vi "_is.vi"(8 "error in (no error)":errorcluster, 11 "Config Plugin in":refnum<class "Config Plugin.lvclass">) -> (0 "error out":errorcluster, 3 "Config Plugin out":refnum<class "Config Plugin.lvclass">)   [LabVIEW 2016, in "Config Plugin.lvlib" / "Config Plugin.lvclass"]
uses:
  <userlib>/Common Components/Config Plugin/Config Plugin.lvclass
panel:
  out "type":string
  # "HW Controller: always shown.\nspecific HW: shown when the hardware class is loaded.\nAbstract Class: for this root class"
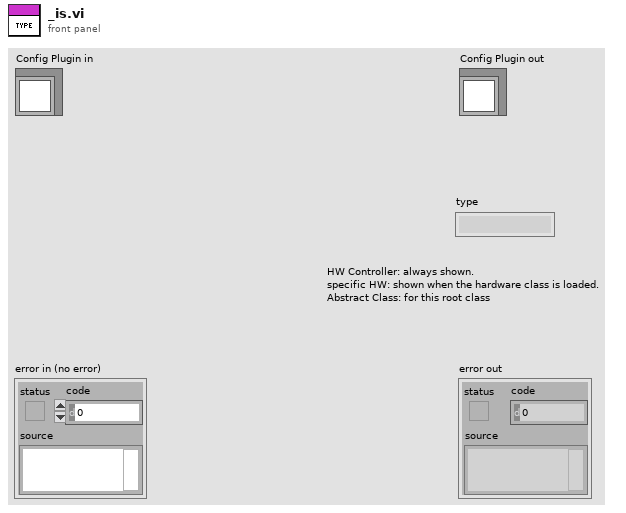
[diagram p1: front panel]
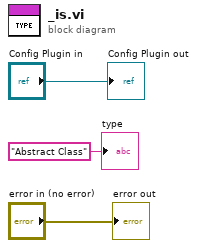
[diagram p0: block diagram]
diagram:
  "error out" <- "error in (no error)"
  "Config Plugin out" <- "Config Plugin in"
  "type" <- "Abstract Class" ("type")
